vi "ziExample-Module-Scope.vi"() -> ()   [LabVIEW 2009]
doc: "Control a Zurich instrument device via the LabOne Labview API. \nRequirements: Zurich Instruments MFLI, HF2 or UHFLI \nThis example shows how to start a scope module and retrieve data.\n\n© Zurich Instruments AG, www.zhinst.com"
uses:
  <instrlib>/Zurich Instruments LabOne/Public/Modules/ziTypeModEnum.ctl
  <instrlib>/Zurich Instruments LabOne/Public/Configure/ziSetValueDouble.vi
  <instrlib>/Zurich Instruments LabOne/Public/Modules/ziModSetValueDoubleArray.vi
  <instrlib>/Zurich Instruments LabOne/Public/Configure/ziGetValueString.vi
  <instrlib>/Zurich Instruments LabOne/Public/Configure/ziSetValueDoubleArray.vi
  <instrlib>/Zurich Instruments LabOne/Public/Modules/ziModGetScopeWave.vi
  <instrlib>/Zurich Instruments LabOne/Public/Modules/ziModSetValueDouble.vi
  <instrlib>/Zurich Instruments LabOne/Zurich Instruments LabOne.lvlib
panel:
  in  "segmentedcount":i32 caption="segmented count"
  in  "segmented":bool
  out "?":sgl[][](graph)
  in  "mode":u16(ring)=1 items=["Time Domain"=1, "Freq Domain FFT"=3]
  in  "stop":bool
  in  "averagerweight":dbl=1.0 caption="averager/weight"
  out "?":cluster{dbl[], "Data Float":sgl[]}[](graph)
  out "Error Out":errorcluster
  in  "Address":string="DEV"
  out "Selected Device":string
  in  "subscribepath":string="scopes/0/wave" caption="Subscribe Path"
  # "Only for non-HF2"
  # "ziExample-SweepModul.vi\nRequirements: HF2LI, UHFLI or MFLI\nsee block diagram for VI description"
  # "Tested Devices:\n- HF2LI\n- UHFLI\n- MFLI"
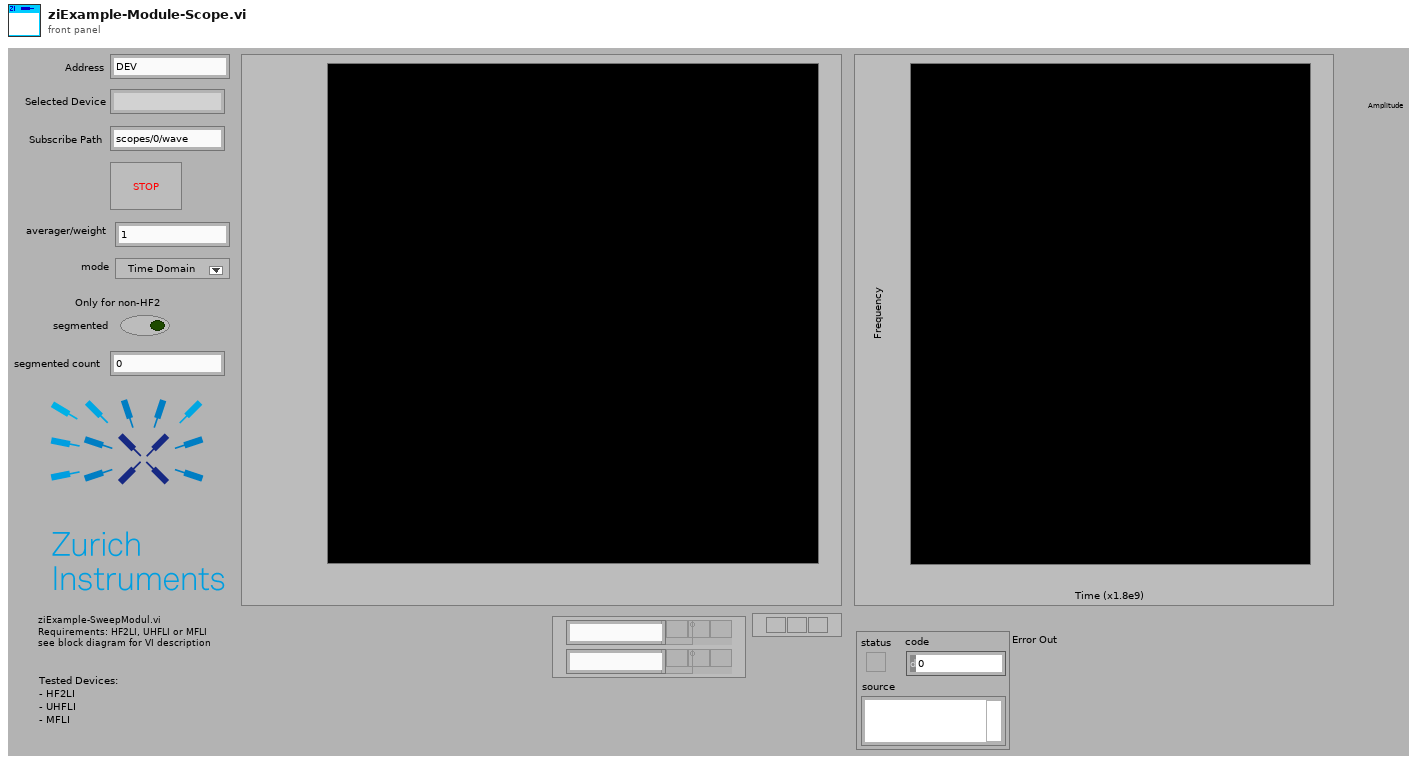
[diagram p1: front panel]
types:
  T1 = typedef "Zurich Instruments LabOne.lvlib/ziTypeModEnum.ctl" = u16
  T2 = typedef "Zurich Instruments LabOne.lvlib/ziTypeHandle.ctl" = cluster{"handleValid":bool, "Conn":u64, "Path Prefix":string, "Handle":u64, "Connected":bool, "Clockbase(s)":dbl}
  T3 = typedef "Zurich Instruments LabOne.lvlib/ziTypeModHandle.ctl" = cluster{"handleValid":bool, "Conn":u64, "ModHandle":u64, "moduleID":string, "Path Prefix":string}
  T4 = typedef "Zurich Instruments LabOne.lvlib/ziTypeModResults.ctl" = cluster{"PathArray":string[], "ValueType":T5, "NoOfResults":u64, "ziGenericHeader":T6[]}
  T5 = typedef "Zurich Instruments LabOne.lvlib/ziTypePollType.ctl" = enum16{"NONE", "DOUBLE_DATA", "INTEGER_DATA", "DEMOD_SAMPLE", "SCOPE_WAVE_HF2", "AUXIN_SAMPLE", "DIO_SAMPLE", "BYTE_ARRAY", "PWA_WAVE", "9", "10", "11", "12", "13", "14", "15", "TREE_CHANGE_DEPRI", "17", "ERROR", "19", "20", "21", "22", "23", "24", "25", "26", "27", "28", "29", "30", "31", "DOUBLE_DATA_TS", "INTEGER_DATA_TS", "34", "SCOPE_WAVE", "SCOPE_WAVE_EX", "37", "BYTE_ARRAY_TS", "39", "40", "41", "42", "43", "44", "45", "CNT_DATA", "47", "TREE_CHANGE", "49", "50", "51", "52", "53", "54", "55", "56", "57", "58", "59", "60", "61", "62", "63", "SWEEPER_DATA", "SPECTRUM_DATA", "ADVISOR_DATA", "VECTOR_DATA", "IMP_DATA"}
  T6 = typedef "Zurich Instruments LabOne.lvlib/ziTypeModGenericHeader.ctl" = cluster{"HeaderType":enum8{"HEADER_TYPE_NONE", "HEADER_TYPE_SWTRIGGER", "HEADER_TYPE_SWEEPER"}, "SampleFormat":u8, "SystemTime":timestamp, "CreatedTimeStamp":u64, "ChangedTimeStamp":u64, "Flags":u32, "ChunkSizeBytes":u64, "Name":string, "Status":u32, "GroupIndex":u32, "Color":u32, "ActiveRow":u32, "TriggerNumber":u64, "GridRows":u32, "GridCols":u32, "GridMode":u32, "GridOperation":u32, "GridDirection":u32, "GridRepetitions":u32, "GridColDelta":dbl, "GridColOffset":dbl, "GridRowDelta":dbl, "GridRowOffset":dbl, "Bandwidth":dbl, "Center":dbl, "Nenbw":dbl}
  T7 = typedef "Zurich Instruments LabOne.lvlib/ziTypeScopeWaveGrid.ctl" = cluster{"Timestamp (ticks)":u64, "Timestamp Trigger (ticks)":u64, "dt (s)":dbl, "Channel Enable":u8[], "Channel Input":enum8{"Signal Input 1", "Signal Input 2", "Trigger Input 1", "Trigger Input 2", "Aux Output 1", "Aux Output 2", "Aux Output 3", "Aux Output 4", "Aux Input 1", "Aux Input 2"}[], "Trigger Enable":u64, "Trigger Input":u64, "Channel BW Limit":u8[], "Channel Math":u8[], "Channel Scaling":sgl[], "Sequence Number":u32, "Segment Number":u32, "Block Number":u32, "Data Transfer Mode":enum8{"Single Transfer", "Block Transfer", "Continuous Transfer", "FFT Single Transfer"}, "Block Marker":enum8{"None", "End of Block"}, "Flags":u8, "Sample Format":enum8{"Int16", "Int32", "Float32", "reserved", "Int16 Interleaved", "Int32 Interleaved", "Float32 Interleaved"}, "Sample Count":u32, "Channel Offset":dbl[], "Data Int16":i16[][], "Data Int32":i32[][], "Data Float":sgl[][], "Total Samples":u32}
  T8 = typedef "Zurich Instruments LabOne.lvlib/ziTypeScopeWave.ctl" = cluster{"Timestamp (ticks)":u64, "Timestamp Trigger (ticks)":u64, "dt (s)":dbl, "Channel Enable":u8[], "Channel Input":enum8{"Signal Input 1", "Signal Input 2", "Trigger Input 1", "Trigger Input 2", "Aux Output 1", "Aux Output 2", "Aux Output 3", "Aux Output 4", "Aux Input 1", "Aux Input 2"}[], "Trigger Enable":u64, "Trigger Input":u64, "Channel BW Limit":u8[], "Channel Math":u8[], "Channel Scaling":sgl[], "Sequence Number":u32, "Segment Number":u32, "Block Number":u32, "Data Transfer Mode":enum8{"Single Transfer", "Block Transfer", "Continuous Transfer", "FFT Single Transfer"}, "Block Marker":enum8{"None", "End of Block"}, "Flags":u8, "Sample Format":enum8{"Int16", "Int32", "Float32", "reserved", "Int16 Interleaved", "Int32 Interleaved", "Float32 Interleaved"}, "Sample Count":u32, "Channel Offset":dbl[], "Data Int16":i16[], "Data Int32":i32[], "Data Float":sgl[], "Total Samples":u64}
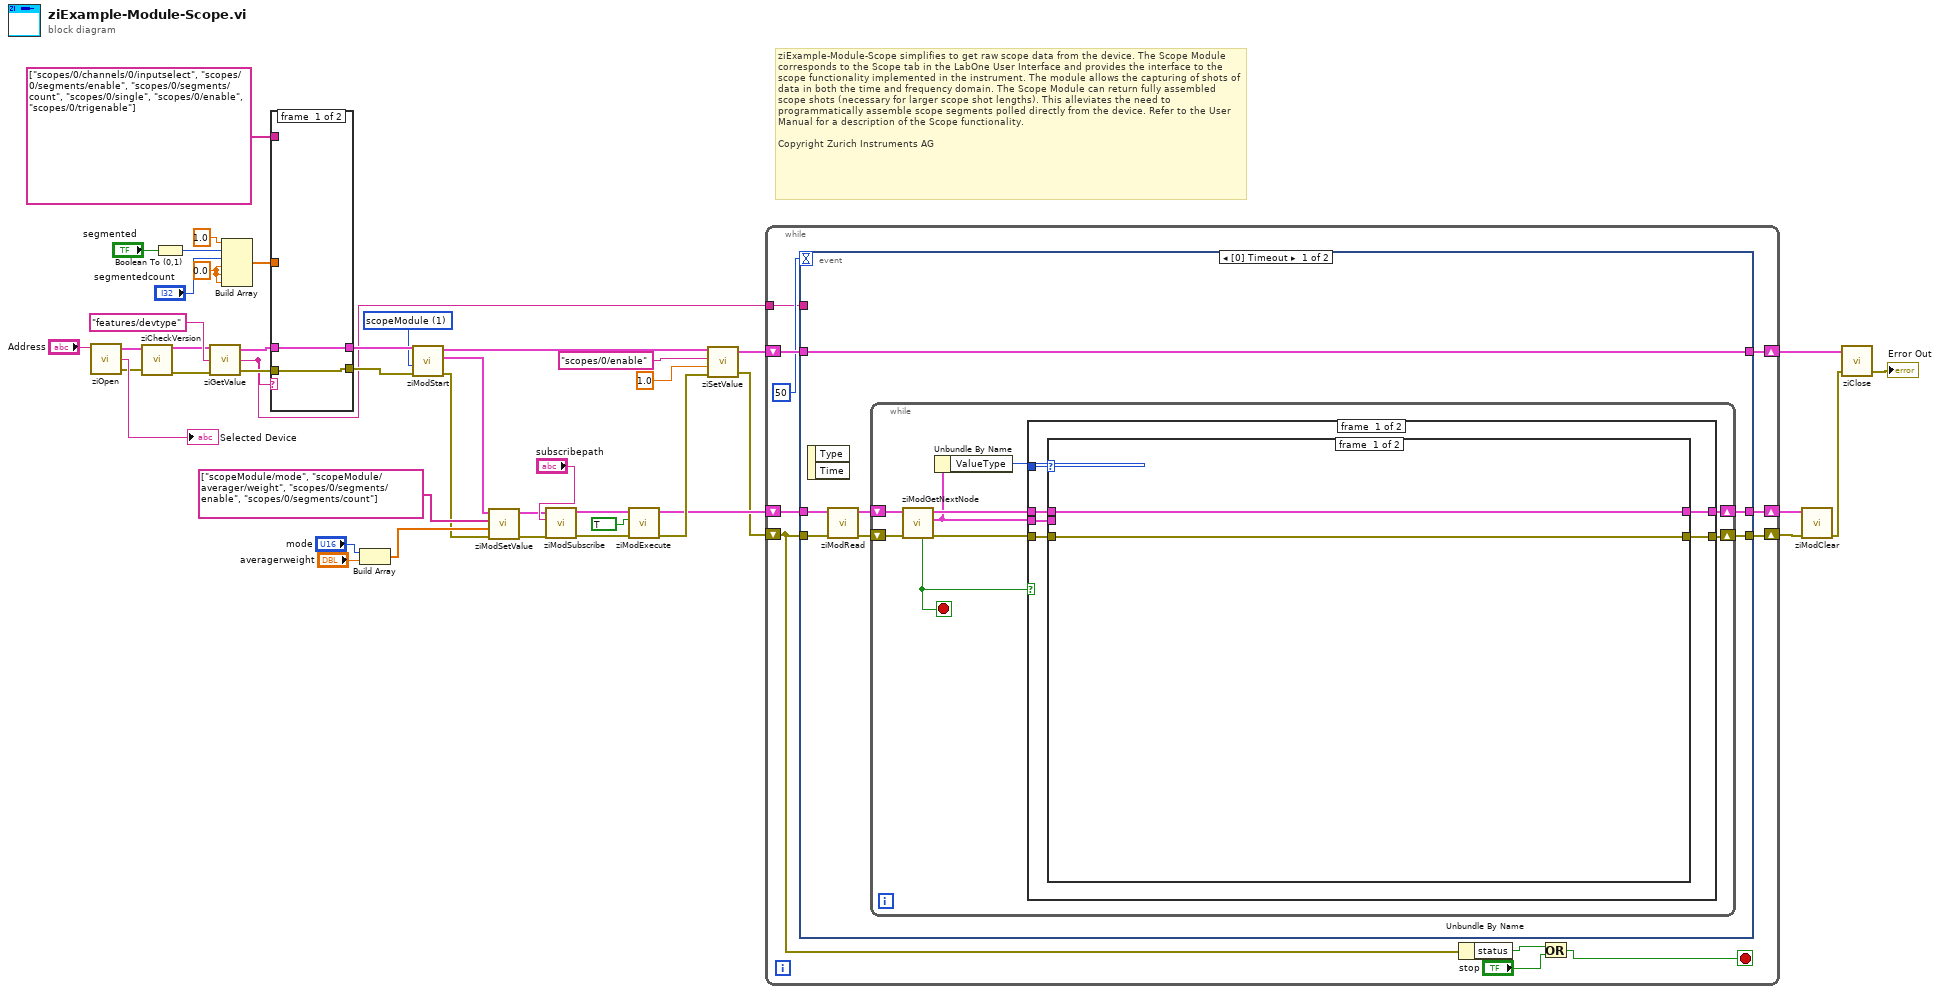
[diagram p0: block diagram]
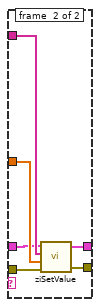
[diagram p2: hidden frame]
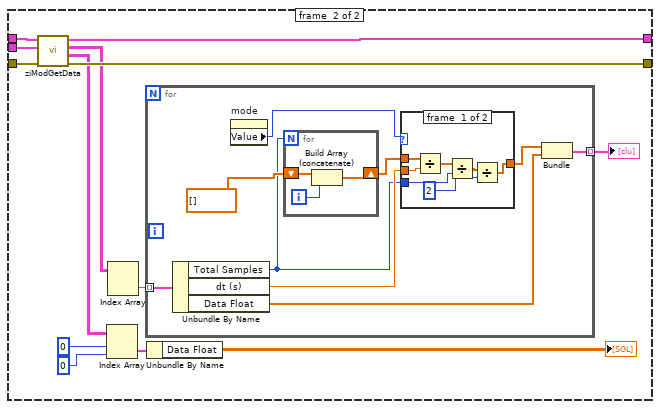
[diagram p3: hidden frame]
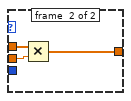
[diagram p4: hidden frame]
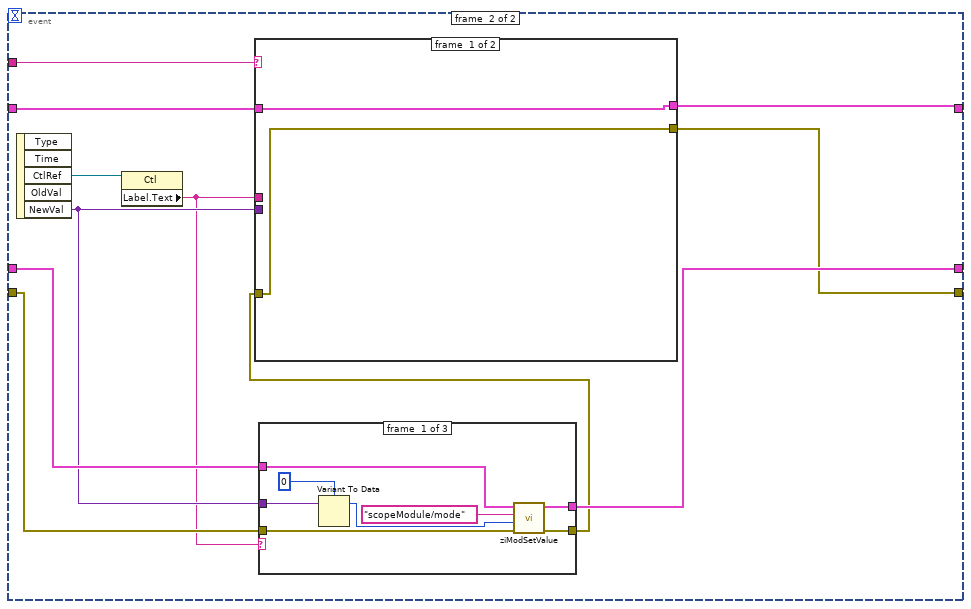
[diagram p6: hidden frame]
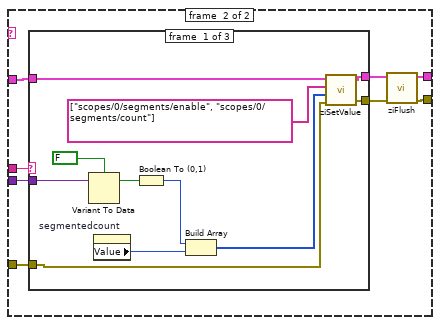
[diagram p7: hidden frame]
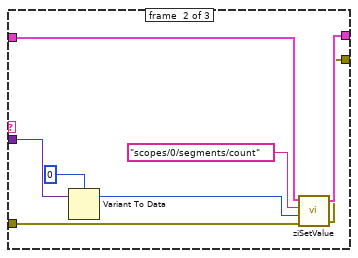
[diagram p8: hidden frame]
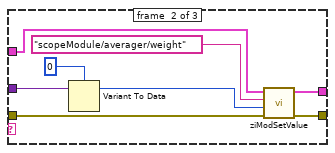
[diagram p10: hidden frame]
diagram:
  w1 = T1 1 items=["sweep", "scopeModule", "dataAcquisitionModule", "pidAdvisor", "awgModule", "impedanceModule", "multiDeviceSyncModule", "zoomFFT", "trigger", "deviceSettings", "record"] ("module Id")
  w7 = 0.0 ("element")
  # "ziExample-Module-Scope simplifies to get raw scope data from the device. The Scope Module corresponds to the Scope tab in the LabOne User Interface and provides the interface to the scope functionality implemented in the instrument. The module allows the capturing of shots of data in both the time and frequency domain. The Scope Module can return fully assembled scope shots (necessary for larger scope shot lengths). This alleviates the need to programmatically assemble scope segments polled directly from the device. Refer to the User Manual for a description of the Scope functionality.\n\nCopyright Zurich Instruments AG"
  n1 = call <instrlib>:"ziOpen.vi"("Address"="Address") -> ("Error Out"=w4:errorcluster, "Selected Device"=→"Selected Device":string, "HandleOut"=w5:T2)  [unwired: 1 in, 2 out]
  n2 = call <instrlib>:"ziCheckVersion.vi"("Handle In"=w5, "Error In"=w4) -> ("Handle Out"=w2:T2, "Error Out"=w3:errorcluster)  [unwired: 11 in, 1 out]
  n3 = Boolean To (0,1)(Boolean="segmented") -> (0, 1=w22:i16)
  n4 = call-poly <instrlib>:"ziGetValue.vi"("error in"=w3, "Path"="features/devtype", "Handle In"=w2) -> ("error out"=w10:errorcluster, "Value"=w9:string, "Handle Out"=w11:T2)
  n5 = Build Array(1.0 ("element"), w22, "segmentedcount", w7, w7, w7) -> (w24:dbl[])
  n6 = case shown="Default" w9 {
    tunnel: [w45 w52] -> w42
    tunnel: string[] ["scopes/0/channels/0/inputselect", "scopes/0/segments/enable", "scopes/0/segments/count", "scopes/0/single", "scopes/0/enable", "scopes/0/trigenable"] -> [_ w51]
    tunnel: [w46 w50] -> w29
    tunnel: w24 -> [_ w49]
    tunnel: w11 -> [w46 w48]
    tunnel: w10 -> [w45 w47]
    frame #0 {
    }
    frame #1 {
      n7 = call-poly <instrlib>:"ziSetValue.vi"("Error In"=w47, "Values"=w49, "Paths"=w51, "Handle In"=w48) -> ("Error Out"=w52:errorcluster, "Handle Out"=w50:T2)  [unwired: 1 in]
    }
  }
  n8 = Build Array("mode", "averagerweight") -> (w20:dbl[])
  n9 = call <instrlib>:"ziModStart.vi"("Error In"=w42, "module Id"=w1, "Handle In"=w29) -> ("Error Out"=w15:errorcluster, "ModHandle Out"=w16:T3, "Handle Out"=w8:T2)  [unwired: 6 in]
  n10 = call-poly <instrlib>:"ziModSetValue.vi"("Error In"=w15, "Values"=w20, "Paths"=string[] ["scopeModule/mode", "scopeModule/averager/weight", "scopes/0/segments/enable", "scopes/0/segments/count"], "ModHandle In"=w16) -> ("Error Out"=w14:errorcluster, "ModHandle Out"=w13:T3)  [unwired: 6 in]
  n11 = call <instrlib>:"ziModSubscribe.vi"("Error In"=w14, "Path"="subscribepath", "ModHandle In"=w13) -> ("Error Out"=w34:errorcluster, "ModHandle Out"=w35:T3)  [unwired: 6 in]
  n12 = call <instrlib>:"ziModExecute.vi"("Error In"=w34, "Modal (F)"=TRUE ("Modal"), "ziModHandle In"=w35) -> ("Error Out"=w33:errorcluster, "ziModHandle Out"=w28:T3)  [unwired: 5 in, 1 out]
  n13 = call-poly <instrlib>:"ziSetValue.vi"("Error In"=w33, "Value"=1.0, "Path"="scopes/0/enable", "Handle In"=w8) -> ("Error Out"=w27:errorcluster, "Handle Out"=w26:T2)  [unwired: 1 in]
  n14 = while {
    shift-right: [w62] -> w39
    shift-left: w27 -> [w53]
    shift-right: [w61] -> w38
    shift-left: w28 -> [w63]
    shift-right: [w59] -> w25
    shift-left: w26 -> [w60]
    tunnel: w9 -> [w57]
    stop <- w54 stop-if-true
    n15 = event shown="[0] Timeout" {
      selector: _ -> [_ _]
      dyn-events: _ -> [_ _]
      timeout: 50 -> [_ _]
      tunnel: w63 -> [w68 w133]
      tunnel: w53 -> [w67 w134]
      tunnel: [w66 w130] -> w62
      tunnel: [w65 w132] -> w61
      tunnel: w60 -> [w64 w129]
      tunnel: [w64 w131] -> w59
      tunnel: w57 -> [_ w125]
      event #0 {
        n16 = event-data() -> ()  [unwired: 1 in, 2 out]
        n17 = call <instrlib>:"ziModRead.vi"("error in"=w67, "ziModHandle In"=w68) -> ("error out"=w70:errorcluster, "ziModHandle Out"=w69:T3)  [unwired: 8 in]
        n18 = while {
          shift-right: [w78] -> w65
          shift-left: w69 -> [w72]
          shift-right: [w77] -> w66
          shift-left: w70 -> [w73]
          stop <- w71 stop-if-true
          n19 = call <instrlib>:"ziModGetNextNode.vi"("Error In"=w73, "ModHandle In"=w72) -> ("Error Out"=w76:errorcluster, "ModResults"=w74:T4, "ModHandle Out"=w79:T3, "NoData"=w71:bool)  [unwired: 6 in]
          n20 = Unbundle By Name(w74) -> ("ValueType"=w75:T5)
          n21 = case shown="False" w71 {
            tunnel: w79 -> [w85 w123]
            tunnel: [w84 w123] -> w78
            tunnel: [w83 w124] -> w77
            tunnel: w76 -> [w82 w124]
            tunnel: w74 -> [w81 _]
            tunnel: w75 -> [w80 _]
            frame #0 {
              n22 = case shown="\"SCOPE_WAVE_EX\"" w80 {
                tunnel: w85 -> [w87 w97]
                tunnel: w81 -> [_ w100]
                tunnel: w82 -> [w86 w99]
                tunnel: [w86 w98] -> w83
                tunnel: [w87 w96] -> w84
                frame #0 {
                }
                frame #1 {
                  n23 = call-poly <instrlib>:"ziModGetData.vi"("Error In"=w99, "ModResults"=w100, "ModHandle In"=w97) -> ("Error Out"=w98:errorcluster, "ModScopeWaveGrid"=w94:T7[][], "ModScopeWave"=w89:T8[][], "ModHandle Out"=w96:T3)  [unwired: 5 in]
                  n24 = Index Array(array=w94, index (row)=0, index (col)=0 ("disabled index (col)")) -> (element=w90:T7)
                  n25 = Index Array(array=w89) -> (element=w88:T8[])  [unwired: 2 in]
                  n26 = for {
                    tunnel: w88 -> [w109] mode=indexing
                    tunnel: [w107] -> w95 mode=indexing
                    n27 = Unbundle By Name(w109) -> ("Total Samples"=w102:u64, "dt (s)"=w104:dbl, "Data Float"=w106:sgl[])
                    n28 = property on="mode" class="Ring (strict)"() -> ("Value"=w105:u16)  [unwired: 2 in, 2 out]
                    n29 = for {
                      N: w102 -> [_]
                      shift-right: [w121] -> w103
                      shift-left: dbl[] [] -> [w122]
                      i -> [w120]
                      n30 = Build Array (concatenate)(w122, w120) -> (w121:dbl[])
                    }
                    n31 = case shown="1, Default" w105 {
                      tunnel: w104 -> [w116 w119]
                      tunnel: w103 -> [w115 w118]
                      tunnel: w102 -> [w114 _]
                      tunnel: [w110 w117] -> w101
                      frame #0 {
                        n32 = Divide(x=w115, y=w116) -> (x/y=w113:dbl[])
                        n33 = Divide(x=w113, y=w114) -> (x/y=w112:dbl[])
                        n34 = Divide(x=w112, y=2) -> (x/y=w110:dbl[])
                      }
                      frame #1 {
                        n35 = Multiply(x=w118, y=w119) -> (x*y=w117:dbl[])
                      }
                    }
                    n36 = Bundle(w101, "Data Float"=w106) -> (w107:cluster{dbl[], "Data Float":sgl[]})  [unwired: 1 in]
                  }
                  "?" <- w95
                  n37 = Unbundle By Name(w90) -> ("Data Float"=→"?":sgl[][])
                }
              }
            }
            frame #1 {
            }
          }
        }
      }
      event #1 {
        n38 = event-data() -> ("CtlRef"=w135:refnum<vi>, "NewVal"=w127:variant)  [unwired: 1 in, 3 out]
        n39 = property class="Ctl"(reference=w135) -> ("Label.Text"=w126:string)  [unwired: 1 in, 2 out]
        n40 = case shown="\"mode\"" w126 {
          tunnel: w127 -> [w174 w182 _]
          tunnel: w134 -> [w171 w179 w184]
          tunnel: [w170 w178 w184] -> w128
          tunnel: w133 -> [w169 w177 w183]
          tunnel: [w168 w176 w183] -> w132
          frame #0 {
            n41 = Variant To Data(Variant=w174, type=u16 0) -> (data=w172:u16)  [unwired: 1 in, 1 out]
            n42 = call-poly <instrlib>:"ziModSetValue.vi"("Error In"=w171, "Value"=w172, "Path"="scopeModule/mode", "ModHandle In"=w169) -> ("Error Out"=w170:errorcluster, "ModHandle Out"=w168:T3)  [unwired: 6 in]
          }
          frame #1 {
            n43 = Variant To Data(Variant=w182, type=0) -> (data=w180:i32)  [unwired: 1 in, 1 out]
            n44 = call-poly <instrlib>:"ziModSetValue.vi"("Error In"=w179, "Value"=w180, "Path"="scopeModule/averager/weight", "ModHandle In"=w177) -> ("Error Out"=w178:errorcluster, "ModHandle Out"=w176:T3)  [unwired: 6 in]
          }
          frame #2 {
          }
        }
        n45 = case shown="Default" w125 {
          tunnel: [w136 w145] -> w131
          tunnel: [w137 w144] -> w130
          tunnel: w129 -> [w136 w142]
          tunnel: w128 -> [w137 w141]
          tunnel: w127 -> [_ w140]
          tunnel: w126 -> [_ w139]
          frame #0 {
          }
          frame #1 {
            n46 = case shown="\"segmented\"" w139 {
              tunnel: w140 -> [w156 w164 _]
              tunnel: w142 -> [w153 w161 w166]
              tunnel: [w152 w160 w166] -> w143
              tunnel: w141 -> [w151 w159 w165]
              tunnel: [w150 w158 w165] -> w138
              frame #0 {
                n47 = Variant To Data(Variant=w156, type=FALSE ("segmented 2")) -> (data=w154:bool)  [unwired: 1 in, 1 out]
                n48 = property on="segmentedcount" class="DigNum (strict)"() -> ("Value"=w146:i32)  [unwired: 2 in, 2 out]
                n49 = Boolean To (0,1)(Boolean=w154) -> (0, 1=w148:i16)
                n50 = Build Array(w148, w146) -> (w147:i32[])
                n51 = call-poly <instrlib>:"ziSetValue.vi"("Error In"=w151, "Values"=w147, "Paths"=string[] ["scopes/0/segments/enable", "scopes/0/segments/count"], "Handle In"=w153) -> ("Error Out"=w150:errorcluster, "Handle Out"=w152:T2)  [unwired: 1 in]
              }
              frame #1 {
                n52 = Variant To Data(Variant=w164, type=0) -> (data=w163:i32)  [unwired: 1 in, 1 out]
                n53 = call-poly <instrlib>:"ziSetValue.vi"("Error In"=w159, "Value"=w163, "Path"="scopes/0/segments/count", "Handle In"=w161) -> ("Error Out"=w158:errorcluster, "Handle Out"=w160:T2)  [unwired: 1 in]
              }
              frame #2 {
              }
            }
            n54 = call <instrlib>:"ziFlush.vi"("error in"=w138, "Handle In"=w143) -> ("error out"=w144:errorcluster, "Handle Out"=w145:T2)  [unwired: 8 in]
          }
        }
      }
    }
    n55 = Unbundle By Name(w53) -> ("status"=w56:bool)
    n56 = Or(x=w56, y="stop") -> (x .or. y?=w54:bool)
  }
  n57 = call <instrlib>:"ziModClear.vi"("Error In"=w39, "ziModHandle In"=w38) -> ("Error Out"=w44:errorcluster)  [unwired: 7 in, 1 out]
  n58 = call <instrlib>:"ziClose.vi"("Error In"=w44, "Handle In"=w25) -> ("Error Out"=→"Error Out":errorcluster)  [unwired: 2 in, 1 out]
